vi "Command Interpreter.vi"(10 "Command":string, 11 "L1-2 Q":refnum<queue>) -> (0 "error out":errorcluster, 3 "queue out":refnum<queue>)   [LabVIEW 2019]
uses:
  main queue data type.ctl
  top level commands.ctl
  Robot Movement Command Interpreter - to rubix.vi
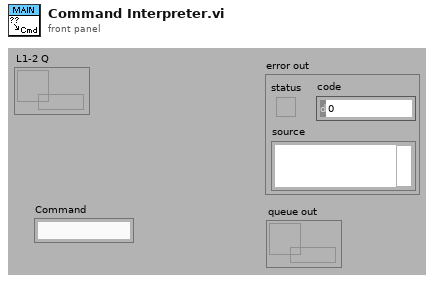
[diagram p1: front panel]
types:
  T1 = typedef "main queue data type.ctl" = cluster{"Command":T2, "Data":variant}
  T2 = typedef "top level commands.ctl" = enum16{"Idle", "Set Cube Orientation", "Get Cube Orientation", "Go to Face", "Solve", "Test", "Randomize", "Game Play Type", "Stop", "rotate Cube"}
  T3 = typedef "facet and command.ctl" = cluster{"Rotate command":T4, "Facet to act on":u8}
  T4 = typedef "Cube Data Ops.ctl" = enum16{"Initialize", "Set Rubix Ref Array", "Set Rubix Text Array", "Set Current Face", "Get Rubix Text Array", "Generate Rubix Array", "Get Rubix array", "Get Facets to move", "Randomize", "Top row left", "Top row right", "Middle row left", "Middle row right", "Bottom row left", "Bottom row right", "Left column up", "Left column down", "Middle column up", "Middle column down", "Right column up", "Right column down", "Face ccw", "Face cw"}
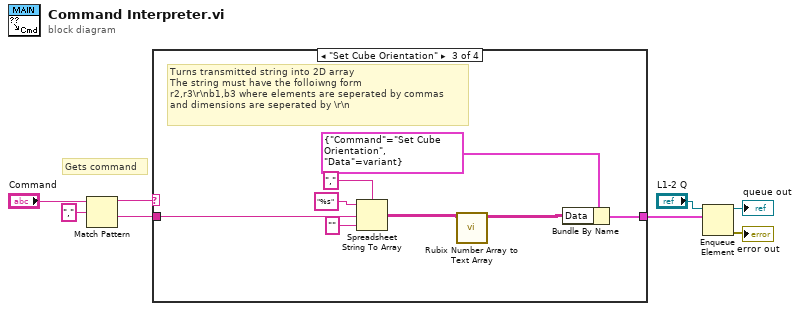
[diagram p0: block diagram]
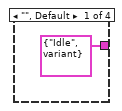
[diagram p2: hidden frame]
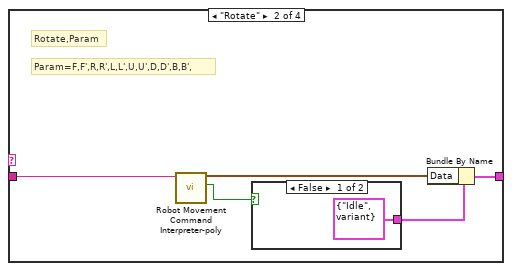
[diagram p3: hidden frame]
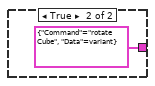
[diagram p4: hidden frame]
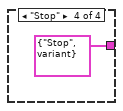
[diagram p5: hidden frame]
diagram:
  # "Gets command"
  n1 = Match Pattern(string="Command", regular expression=",") -> (before substring=w6:string, after substring=w4:string)  [unwired: 1 in, 2 out]
  n2 = case shown="\"Set Cube Orientation\"" w6 {
    tunnel: [T1 {"Command"=enum."Idle", "Data"=variant} ("element") w14 w23 T1 {"Command"=enum."Stop", "Data"=variant} ("element")] -> w8
    tunnel: w4 -> [_ w12 w19 _]
    frame "", Default {
    }
    frame "Rotate" {
      # "Param=F,F',R,R',L,L',U,U',D,D',B,B',"
      # "Rotate,Param"
      n3 = call-poly "Robot Movement Command Interpreter-poly.vi"("Rbt Cmd"=w12) -> ("Valid  Cmd?"=w10:bool, "Rubix Cmd"=w11:T3)  [unwired: 8 in, 1 out]
      n4 = case shown="False" w10 {
        tunnel: [T1 {"Command"=enum."Idle", "Data"=variant} ("element") T1 {"Command"=enum."rotate Cube", "Data"=variant} ("element")] -> w13
        frame False {
        }
        frame True {
        }
      }
      n5 = Bundle By Name(cluster=w13, "Data"=w11) -> (w14:T1)
    }
    frame "Set Cube Orientation" {
      # "Turns transmitted string into 2D array\nThe string must have the folloiwng form\nr2,r3\\r\\nb1,b3 where elements are seperated by commas\nand dimensions are seperated by \\r\\n"
      n6 = Spreadsheet String To Array(delimiter (Tab)=",", format string="%s", spreadsheet string=w19, array type (2D Dbl)="" ("regular expression")) -> (array=w18:string[][])
      n7 = call "Rubix Number Array to Text Array.vi"("Cube Orientation"=w18) -> ("Text Array"=w17:string[][])  [unwired: 10 in]
      n8 = Bundle By Name(cluster=T1 {"Command"=enum."Set Cube Orientation", "Data"=variant} ("element"), "Data"=w17) -> (w23:T1)
    }
    frame "Stop" {
    }
  }
  n9 = Enqueue Element(queue="L1-2 Q", element=w8) -> (queue out=→"queue out":refnum<queue>, error out=→"error out":errorcluster)  [unwired: 2 in, 1 out]
